vi "CAN open.vi"(5 "CAN Baudrate":u16(ring)=5120 items=["10 kBd"=7217, "20 kBd"=7192, "50 kBd"=7177, "100 kBd"=7172, "125 kBd "=7171, "250 kBd"=7169, "500 kBd"=7168, "800 kBd"=5632, "1000 kBd "=5120], 6 "CAN Number":u32(ring) items=["CAN 0", "CAN 1"]) -> (0 "CAN Control Handle":u32=149880912, 1 "Device Handle":u32=149815376, 2 "CAN Channel Handle":u32=149946448, 3 "Channel is active":bool, 4 "CAN controller is started":bool)   [LabVIEW 2011]
panel:
  out "BTR 1":u8=20 format="%02x"
  out "BTR 0":u8 format="%02x"
  in  "Operating Mode":T1={"standard"=TRUE, "extended"=TRUE, "errorframes"=FALSE, "listenonly"=FALSE, "lowspeed"=FALSE}
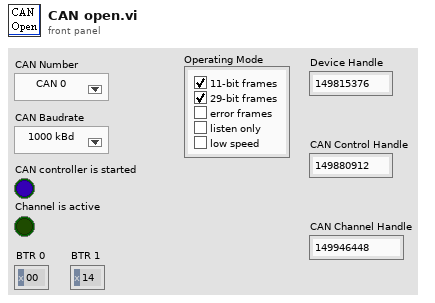
[diagram p1: front panel]
types:
  T1 = cluster{"standard":bool, "extended":bool, "errorframes":bool, "listenonly":bool, "lowspeed":bool}
  T2 = cluster{"Unique VCI Object ID":cluster{"Low Part":u32, "High Part":u32}, "Driver Version":cluster{"Major":u16, "Minor":u16}, "Hardware Version":cluster{"Major":u16, "Minor":u16}, "Device Class ID":cluster{"D1":u32, "D2":u16, "D3":u16, "D41":u8, "D42":u8, "D43":u8, "D44":u8, "D45":u8, "D46":u8, "D47":u8, "D48":u8}, "Unique Hardware ID":cluster{"D1":u32, "D2":u16, "D3":u16, "D41":u8, "D42":u8, "D43":u8, "D44":u8, "D45":u8, "D46":u8, "D47":u8, "D48":u8}, "Description":string, "Manufacturer":string}
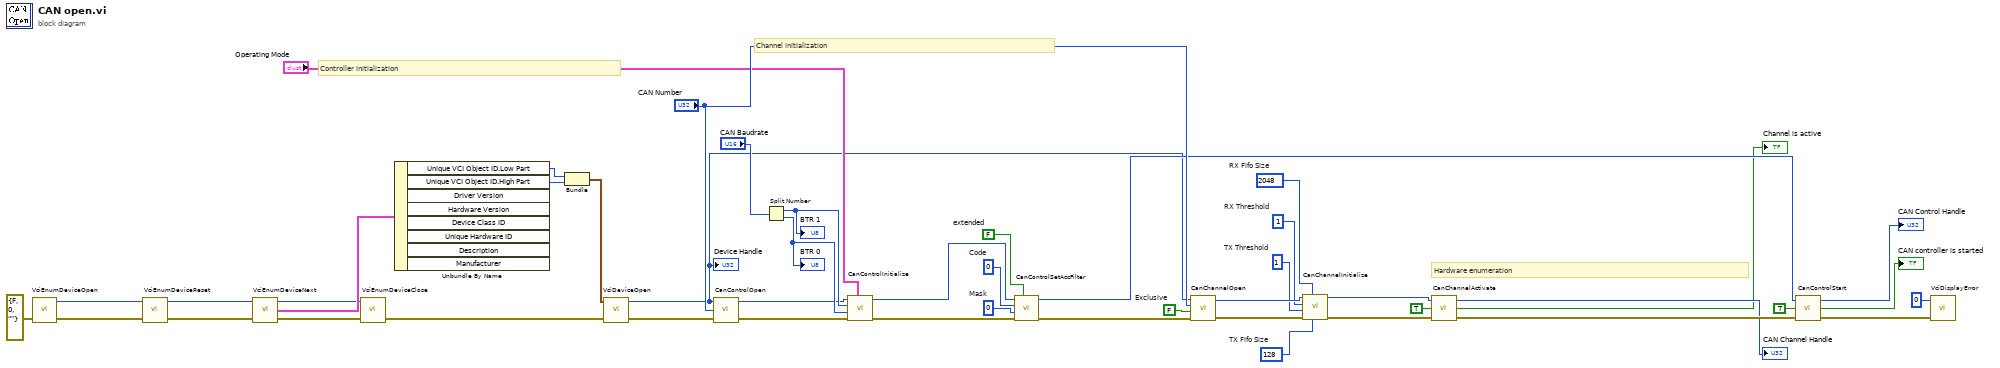
[diagram p0: block diagram]
diagram:
  w33 = u16 128  # TX Fifo Size
  w32 = u16 1  # TX Threshold
  w31 = u16 1  # RX Threshold
  w30 = u16 2048  # RX Fifo Size
  w29 = FALSE  # Exclusive
  w27 = u32 0  # Mask
  w26 = u32 0  # Code
  w25 = FALSE items=["OFF", "ON", "OFF", "ON"]  # extended
  # "Channel initialization"
  # "Controller initialization"
  # "Hardware enumeration"
  n1 = call "VciEnumDeviceOpen.vi"("error in"=errorcluster {"status"=FALSE, "code"=0, "source"=""}) -> ("error out"=w19:errorcluster, "Enum Handle out"=w15:u32)  [unwired: 3 in]
  n2 = call "VciEnumDeviceReset.vi"("error in"=w19, "Enum Handle in"=w15) -> ("error out"=w46:errorcluster, "Enum Handle out"=w16:u32)  [unwired: 2 in]
  n3 = call "VciEnumDeviceNext.vi"("error in"=w46, "Enum Handle in"=w16) -> ("error out"=w6:errorcluster, "Device Info"=w12:T2, "Enum Handle out"=w4:u32)  [unwired: 1 in]
  n4 = call "VciEnumDeviceClose.vi"("error in"=w6, "Enum Handle in"=w4) -> ("error out"=w5:errorcluster)  [unwired: 3 in]
  n5 = Unbundle By Name(w12) -> ("Unique VCI Object ID.Low Part"=w11:u32, "Unique VCI Object ID.High Part"=w17:u32)  [unwired: 6 out]
  n6 = Bundle("Low Part"=w11, "High Part"=w17) -> (w18:cluster{"Low Part":u32, "High Part":u32})  [unwired: 1 in]
  n7 = call "VciDeviceOpen.vi"("error in"=w5, "Device ID"=w18) -> ("error out"=w44:errorcluster, "Device Handle"=w9:u32)  [unwired: 2 in]
  "Device Handle" <- w9
  n8 = call "CanControlOpen.vi"("error in"=w44, "CAN Number"="CAN Number", "Device Handle"=w9) -> ("error out"=w22:errorcluster, "CAN Control Handle"=w10:u32)  [unwired: 1 in]
  n9 = Split Number(x="CAN Baudrate") -> (hi(x)=w43:u8, lo(x)=w42:u8)
  "BTR 0" <- w42
  "BTR 1" <- w43
  n10 = call "CanControlInitialize.vi"("Operating Mode"="Operating Mode", "error in"=w22, "BTR 0"=w42, "BTR 1"=w43, "CAN Control Handle in"=w10) -> ("error out"=w24:errorcluster, "CAN Control Handle out"=w23:u32)  [unwired: 1 in, 1 out]
  n11 = call "CanControlSetAccFilter.vi"("extended"=w25, "error in"=w24, "Mask"=w27, "Code"=w26, "CAN Control Handle in"=w23) -> ("error out"=w28:errorcluster, "CAN Control Handle out"=w37:u32)  [unwired: 2 in]
  n12 = call "CanChannelOpen.vi"("error in"=w28, "Exclusive"=w29, "CAN Number"="CAN Number", "Device Handle"=w9) -> ("error out"=w40:errorcluster, "CAN Channel Handle"=w45:u32)  [unwired: 1 in]
  n13 = call "CanChannelInitialize.vi"("TX Fifo Size"=w33, "RX Fifo Size"=w30, "error in"=w40, "TX Threshold"=w32, "RX Threshold"=w31, "CAN Channel Handle in"=w45) -> ("error out"=w35:errorcluster, "CAN Channel Handle out"=w34:u32)  [unwired: 1 in, 1 out]
  n14 = call "CanChannelActivate.vi"("error in"=w35, "activate"=TRUE, "CAN Channel Handle in"=w34) -> ("error out"=w39:errorcluster, "is active"=→"Channel is active":bool, "CAN Channel Handle out"=→"CAN Channel Handle":u32)
  n15 = call "CanControlStart.vi"("error in"=w39, "start"=TRUE, "CAN Control Handle in"=w37) -> ("error out"=w13:errorcluster, "is started"=→"CAN controller is started":bool, "CAN Control Handle out"=→"CAN Control Handle":u32)
  n16 = call "VciDisplayError.vi"("error in"=w13, "HWND Parent"=u32 0) -> ()  [unwired: 4 in]
